vi "etc_XCITE_GetLogBits.vi"(8 "error in (no error)":errorcluster {"code" format="%x"}) -> (0 "error out":errorcluster {"code" format="%x"}, 3 "bits":u32)   [LabVIEW 2019, in "XCite.lvlib"]
doc: "Sends a command to execute on the slelected X-cite device."
uses:
  XCite.lvlib
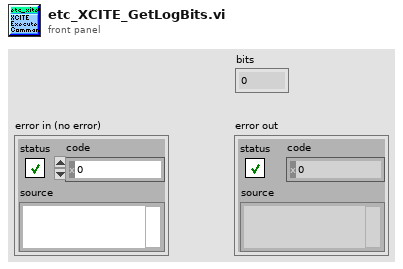
[diagram p1: front panel]
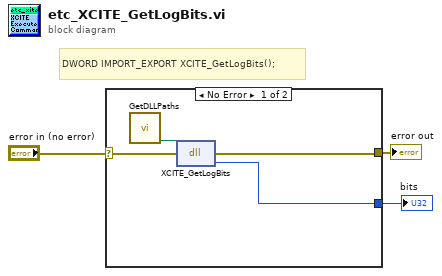
[diagram p0: block diagram]
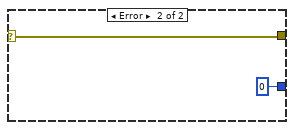
[diagram p2: hidden frame]
diagram:
  # "DWORD IMPORT_EXPORT XCITE_GetLogBits();"
  n1 = case shown="No Error" "error in (no error)" {
    selector: "error in (no error)" -> [w7 w9]
    tunnel: [w4 w9] -> w3
    tunnel: [w5 0 ("return type")] -> w1
    frame No Error {
      n2 = call "GetDLLPaths.vi"() -> ("etc_xcite_path"=w6:path)  [unwired: 8 in, 3 out]
      n3 = dll-call lib="C:/LabVIEWDevFall2024/pco.labview/labview_sdk/runtime/bin64/etc_xcite.dll" fn="XCITE_GetLogBits"(path in=w6, error in=w7) -> (error out=w4:errorcluster, "return type"=w5:u32)  [unwired: 1 in, 1 out]
    }
    frame Error {
    }
  }
  "error out" <- w3
  "bits" <- w1
